vi "TCPSendRec.vi"(0 "TCP Conn":refnum<k5>, 1 "SendLEDRef":refnum<vi>, 2 "RecLEDRef":refnum<vi>, 5 "H2F Frame Ref":refnum<vi>, 11 "error in (no error)":errorcluster) -> (4 "TCP Network Connection out":refnum<k5>, 6 "Bifurcated Recieved Data":T1, 8 "Recieved Frame":string, 10 "TCP Written Bytes":i32, 15 "error out":errorcluster)   [LabVIEW 2018]
uses:
  TypeDefs/recDataClust.ctl
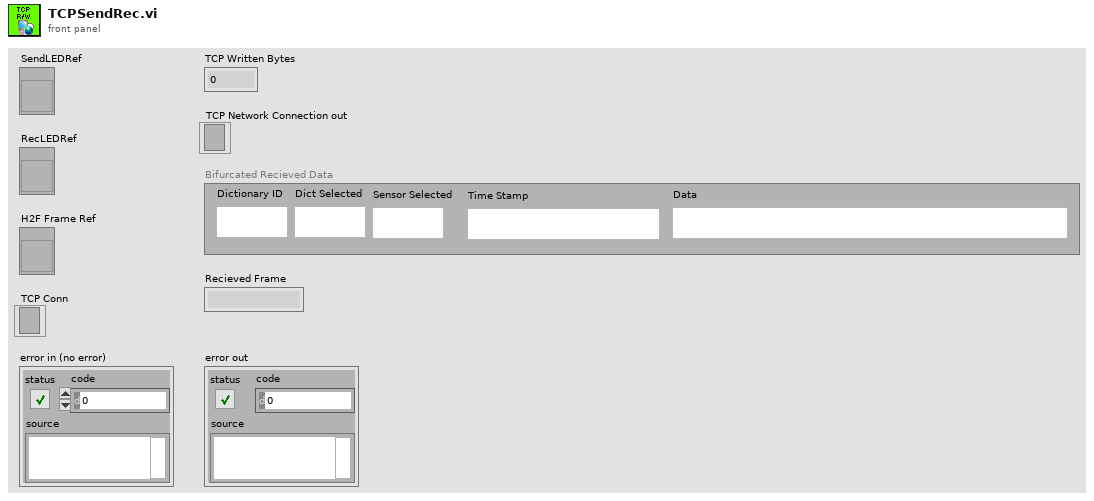
[diagram p1: front panel]
types:
  T1 = typedef "recDataClust.ctl" = cluster{"Dictionary ID":string, "Dict Selected":string, "Sensor Selected":string, "Time Stamp":string, "Data":string}
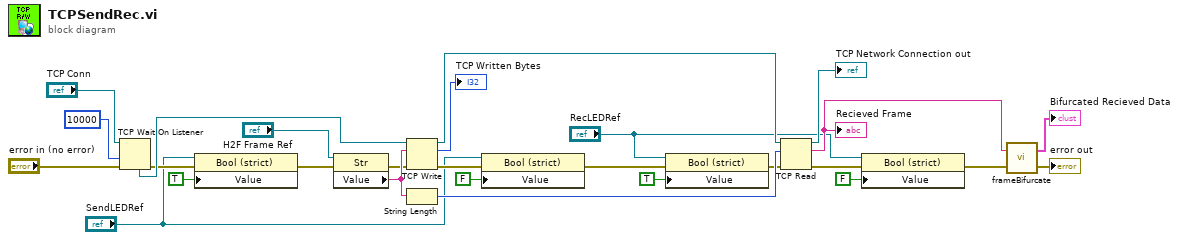
[diagram p0: block diagram]
diagram:
  n1 = TCP Wait On Listener(8:"error in (no error)", 9:10000 ("timeout ms (wait forever: -1)"), 11:"TCP Conn") -> (0:w11:errorcluster, 4:w13:refnum<k5>)  [unwired: 1 in, 3 out]
  n2 = property on="Property Node" class="Bool (strict)"(reference="SendLEDRef", error in=w11, "Value"=TRUE ("Sending Command")) -> (error out=w6:errorcluster)  [unwired: 1 out]
  n3 = property on="Property Node" class="Str"(reference="H2F Frame Ref", error in=w6) -> (error out=w4:errorcluster, "Value"=w27:string)  [unwired: 1 out]
  n4 = TCP Write(connection ID=w13, data in=w27, error in (no error)=w4) -> (connection ID out=w7:refnum<k5>, bytes written=→"TCP Written Bytes":i32, error out=w8:errorcluster)  [unwired: 1 in]
  n5 = String Length(string=w27) -> (length=w26:i32)
  n6 = property on="Property Node" class="Bool (strict)"(reference="SendLEDRef", error in=w8, "Value"=FALSE ("Sending Command")) -> (error out=w14:errorcluster)  [unwired: 1 out]
  n7 = property on="Property Node" class="Bool (strict)"(reference="RecLEDRef", error in=w14, "Value"=TRUE ("Sending Command")) -> (error out=w15:errorcluster)  [unwired: 1 out]
  n8 = TCP Read(connection ID=w7, bytes to read=w26, error in (no error)=w15) -> (connection ID out=→"TCP Network Connection out":refnum<k5>, data out=w23:string, error out=w17:errorcluster)  [unwired: 2 in]
  "Recieved Frame" <- w23
  n9 = property on="Property Node" class="Bool (strict)"(reference="RecLEDRef", error in=w17, "Value"=FALSE ("Sending Command")) -> (error out=w22:errorcluster)  [unwired: 1 out]
  n10 = call "frameBifurcate.vi"("error in (no error)"=w22, "H2F Frame"=w23) -> ("error out"=→"error out":errorcluster, "Bifurcated Recieved Data"=→"Bifurcated Recieved Data":T1)
